vi "Int_Float.vi"(2 "2 Int in":i32 format="%.0x", 3 "1 Float in":sgl min=0 format="%#_6f") -> (0 "2 float out":ext, 1 "1 Int out":i32 format="%.0x")   [LabVIEW 2017]
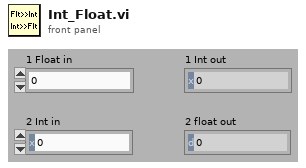
[diagram p1: front panel]
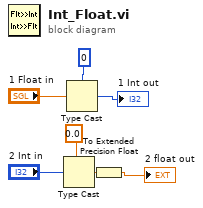
[diagram p0: block diagram]
diagram:
  n1 = Type Cast(type=sgl 0.0, x="2 Int in") -> (*(type *) &x=w5:sgl)
  n2 = Type Cast(type=0 ("Numeric 2"), x="1 Float in") -> (*(type *) &x=→"1 Int out":i32)
  n3 = To Extended Precision Float(1:w5) -> (0:→"2 float out":ext)
